vi "validate line configuration.vi"(7 "Module Config":refnum<class "Daqmx Module configuration.lvclass">, 11 "Mappings in":T1={"Line"={"Channel Array"=[], "Physical Channel"="", "Measurement Type"=enum."Digital Input", "Parameters"={"Digital Config"={"Invert Lines?"=FALSE}, "Voltage Config"={"Maximum Value (V)"=5.0, "Minimum Value (V)"=-5.0, "in terminal configuration (V)"=-1, "out terminal configuration (V)"=-1}, "Current Config"={"Maximum Value (A)"=0.02, "Minimum Value (A)"=0.0, "shunt resistor location"=-1, "input terminal configuration (C)"=-1, "external shunt resistor value"=249.0}, "RTD Config"={"Maximum Value (°C)"=100.0, "Minimum Value (°C)"=0.0, "resistance configuration"=2, "r0"=100.0, "current excitation value"=0.0025, "rtd type"=10137, "current excitation source"=10167}, "Thermocouple Config"={"Minimum Value (C)"=0.0, "Maximum Value (C)"=100.0, "thermocouple type"=10072, "cjc source"=10116, "cjc value"=25.0}, "Strain Config"={"Maximum Value"=0.001, "Minimum Value"=-0.001, "bridge information"={"strain configuration"=10183, "lead wire resistance"=0.0, "initial bridge voltage"=0.0, "voltage excitation source"=10200, "voltage excitation value"=2.5}, "strain gage information"={"gage factor"=2.0, "nominal gage resistance"=350.0, "poisson ratio"=0.3}}, "PWM Config"={"Idle State"=FALSE}}}, "Maps"=[]} {"Line"."Parameters"."Voltage Config"."out terminal configuration (V)" items=["Default"=-1, "RSE"=10083, "Differential"=10106, "Pseudodifferential"=12529]; "Line"."Parameters"."Voltage Config"."in terminal configuration (V)" items=["Default"=-1, "RSE"=10083, "NRSE"=10078, "Differential"=10106, "Pseudodifferential"=12529]; "Line"."Parameters"."Current Config"."shunt resistor location" items=["default"=-1, "Internal"=10200, "External"=10167]; "Line"."Parameters"."Current Config"."input terminal configuration (C)" items=["default"=-1, "RSE"=10083, "NRSE"=10078, "Differential"=10106, "Pseudodifferential"=12529]; "Line"."Parameters"."RTD Config"."resistance configuration" items=["2-Wire"=2, "3-Wire"=3, "4-Wire"=4]; "Line"."Parameters"."RTD Config"."rtd type" items=["Pt3750"=12481, "Pt3851"=10071, "Pt3911"=12482, "Pt3916"=10069, "Pt3920"=10053, "Pt3928"=12483, "Custom"=10137]; "Line"."Parameters"."RTD Config"."current excitation source" items=["Internal"=10200, "External"=10167, "None"=10230]; "Line"."Parameters"."Thermocouple Config"."thermocouple type" items=["J"=10072, "K"=10073, "N"=10077, "R"=10082, "S"=10085, "T"=10086, "B"=10047, "E"=10055]; "Line"."Parameters"."Thermocouple Config"."cjc source" items=["Built-In"=10200, "Constant Value"=10116, "Channel"=10113]; "Line"."Parameters"."Strain Config"."bridge information"."strain configuration" items=["Full Bridge I"=10183, "Full Bridge II"=10184, "Full Bridge III"=10185, "Half Bridge I"=10188, "Half Bridge II"=10189, "Quarter Bridge I"=10271, "Quarter Bridge II"=10272]; "Line"."Parameters"."Strain Config"."bridge information"."voltage excitation source" items=["Internal"=10200, "External"=10167, "None"=10230]}) -> (1 "valid?":bool, 2 "errors":string, 3 "Mappings out":T1={"Line"={"Channel Array"=[], "Physical Channel"="", "Measurement Type"=enum."Digital Input", "Parameters"={"Digital Config"={"Invert Lines?"=FALSE}, "Voltage Config"={"Maximum Value (V)"=5.0, "Minimum Value (V)"=-5.0, "in terminal configuration (V)"=-1, "out terminal configuration (V)"=-1}, "Current Config"={"Maximum Value (A)"=0.02, "Minimum Value (A)"=0.0, "shunt resistor location"=-1, "input terminal configuration (C)"=-1, "external shunt resistor value"=249.0}, "RTD Config"={"Maximum Value (°C)"=100.0, "Minimum Value (°C)"=0.0, "resistance configuration"=2, "r0"=100.0, "current excitation value"=0.0025, "rtd type"=10137, "current excitation source"=10167}, "Thermocouple Config"={"Minimum Value (C)"=0.0, "Maximum Value (C)"=100.0, "thermocouple type"=10072, "cjc source"=10116, "cjc value"=25.0}, "Strain Config"={"Maximum Value"=0.001, "Minimum Value"=-0.001, "bridge information"={"strain configuration"=10183, "lead wire resistance"=0.0, "initial bridge voltage"=0.0, "voltage excitation source"=10200, "voltage excitation value"=2.5}, "strain gage information"={"gage factor"=2.0, "nominal gage resistance"=350.0, "poisson ratio"=0.3}}, "PWM Config"={"Idle State"=FALSE}}}, "Maps"=[]} {"Line"."Parameters"."Voltage Config"."out terminal configuration (V)" items=["Default"=-1, "RSE"=10083, "Differential"=10106, "Pseudodifferential"=12529]; "Line"."Parameters"."Voltage Config"."in terminal configuration (V)" items=["Default"=-1, "RSE"=10083, "NRSE"=10078, "Differential"=10106, "Pseudodifferential"=12529]; "Line"."Parameters"."Current Config"."shunt resistor location" items=["default"=-1, "Internal"=10200, "External"=10167]; "Line"."Parameters"."Current Config"."input terminal configuration (C)" items=["default"=-1, "RSE"=10083, "NRSE"=10078, "Differential"=10106, "Pseudodifferential"=12529]; "Line"."Parameters"."RTD Config"."resistance configuration" items=["2-Wire"=2, "3-Wire"=3, "4-Wire"=4]; "Line"."Parameters"."RTD Config"."rtd type" items=["Pt3750"=12481, "Pt3851"=10071, "Pt3911"=12482, "Pt3916"=10069, "Pt3920"=10053, "Pt3928"=12483, "Custom"=10137]; "Line"."Parameters"."RTD Config"."current excitation source" items=["Internal"=10200, "External"=10167, "None"=10230]; "Line"."Parameters"."Thermocouple Config"."thermocouple type" items=["J"=10072, "K"=10073, "N"=10077, "R"=10082, "S"=10085, "T"=10086, "B"=10047, "E"=10055]; "Line"."Parameters"."Thermocouple Config"."cjc source" items=["Built-In"=10200, "Constant Value"=10116, "Channel"=10113]; "Line"."Parameters"."Strain Config"."bridge information"."strain configuration" items=["Full Bridge I"=10183, "Full Bridge II"=10184, "Full Bridge III"=10185, "Half Bridge I"=10188, "Half Bridge II"=10189, "Quarter Bridge I"=10271, "Quarter Bridge II"=10272]; "Line"."Parameters"."Strain Config"."bridge information"."voltage excitation source" items=["Internal"=10200, "External"=10167, "None"=10230]})   [LabVIEW 2015, in "DAQmx Module editor node.lvclass"]
doc: "This VI validates modifications to the table of lines and returns any errors as strings."
uses:
  DAQmx Module editor node.lvclass
  Mappings.ctl
  <vilib>/NI/Tag Bus Module Framework/channel/TBM channel.lvclass
  module/configuration/Line.ctl
  module/configuration/Measurement Type.ctl
  module/configuration/Parameters.ctl
  Map.ctl
  module/configuration/Daqmx Module configuration.lvclass
  <vilib>/NI/Tag Bus/tag/tag descriptor.lvclass/tag descriptor.ctl
  <vilib>/NI/Tag Bus/tag/read tag name.vi
  <vilib>/NI/Tag Bus/tag/read data type.vi
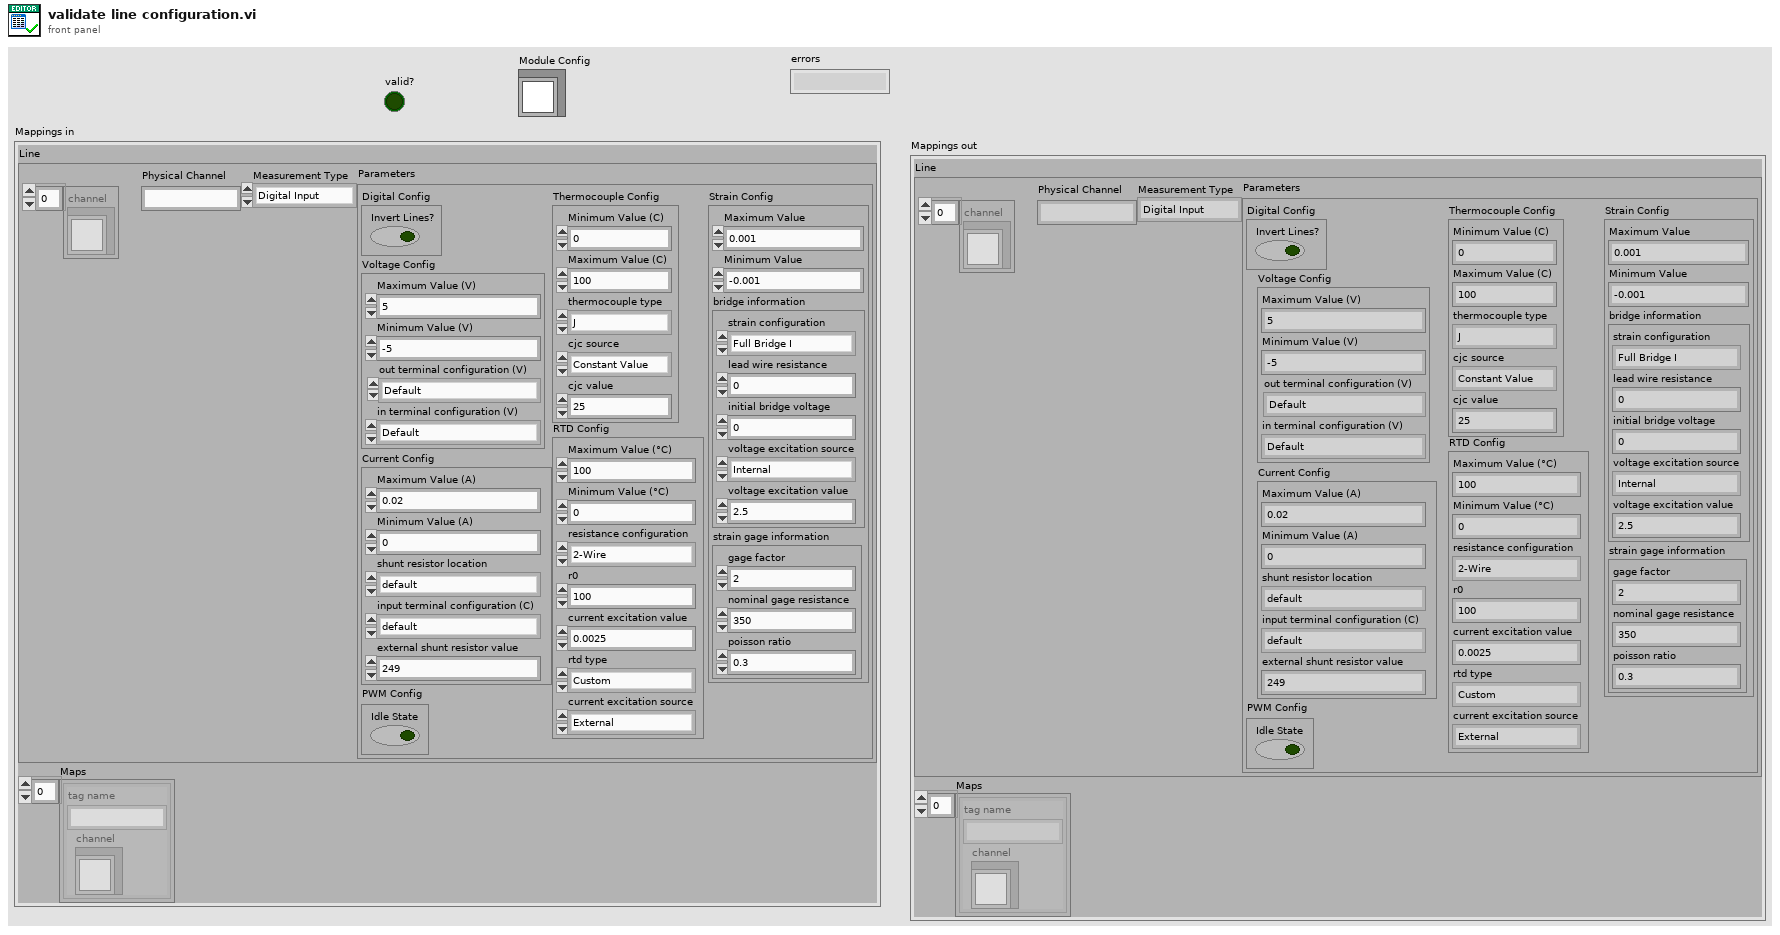
[diagram p1: front panel]
types:
  T1 = typedef "DAQmx Module editor node.lvclass/Mappings.ctl" = cluster{"Line":T2, "Maps":T5[]}
  T2 = typedef "DAQmx Module Configuration.lvclass/Line.ctl" = cluster{"Channel Array":refnum<class "TBM channel.lvclass">[], "Physical Channel":string, "Measurement Type":T3, "Parameters":T4}
  T3 = typedef "DAQmx Module Configuration.lvclass/Measurement Type.ctl" = enum16{"Digital Input", "Digital Output", "Voltage Input", "Voltage Output", "Current Input", "Current Output", "RTD", "Thermocouple", "Strain", "PWM"}
  T4 = typedef "DAQmx Module Configuration.lvclass/Parameters.ctl" = cluster{"Digital Config":cluster{"Invert Lines?":bool}, "Voltage Config":cluster{"Maximum Value (V)":dbl, "Minimum Value (V)":dbl, "in terminal configuration (V)":i32, "out terminal configuration (V)":i32}, "Current Config":cluster{"Maximum Value (A)":dbl, "Minimum Value (A)":dbl, "shunt resistor location":i32, "input terminal configuration (C)":i32, "external shunt resistor value":dbl}, "RTD Config":cluster{"Maximum Value (°C)":dbl, "Minimum Value (°C)":dbl, "resistance configuration":i32, "r0":dbl, "current excitation value":dbl, "rtd type":i32, "current excitation source":i32}, "Thermocouple Config":cluster{"Minimum Value (C)":dbl, "Maximum Value (C)":dbl, "thermocouple type":i32, "cjc source":i32, "cjc value":dbl}, "Strain Config":cluster{"Maximum Value":dbl, "Minimum Value":dbl, "bridge information":cluster{"strain configuration":i32, "lead wire resistance":dbl, "initial bridge voltage":dbl, "voltage excitation source":i32, "voltage excitation value":dbl}, "strain gage information":cluster{"gage factor":dbl, "nominal gage resistance":dbl, "poisson ratio":dbl}}, "PWM Config":cluster{"Idle State":bool}}
  T5 = typedef "DAQmx Module editor node.lvclass/Map.ctl" = cluster{"channel":refnum<class "TBM channel.lvclass">, "tag name":string}
  T6 = typedef "tag bus.lvlib/tag descriptor.lvclass/Data Type.ctl" = enum16{"Double", "Single", "I64", "I32", "I16", "I8", "U64", "U32", "U16", "U8", "Boolean", "String", "Array of Double", "Array of Single", "Array of I64", "Array of I32", "Array of I16", "Array of I8", "Array of U64", "Array of U32", "Array of U16", "Array of U8", "Array of Boolean", "Array of String"}
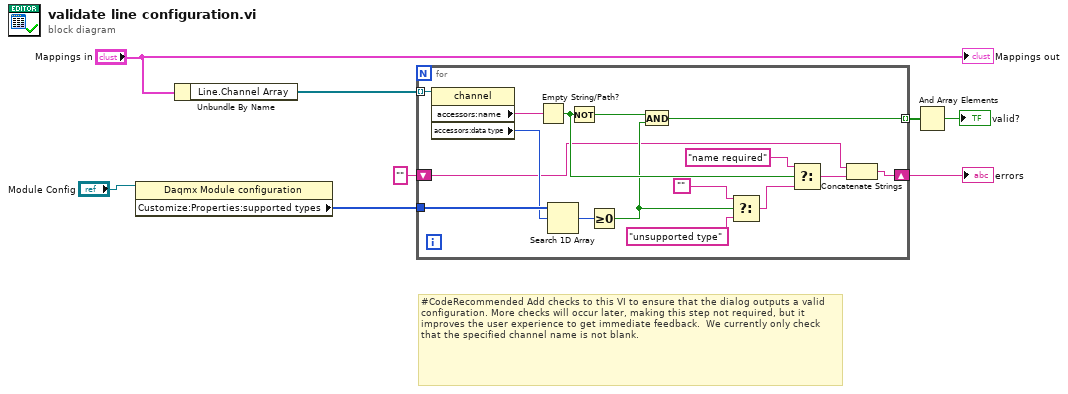
[diagram p0: block diagram]
diagram:
  # "#CodeRecommended Add checks to this VI to ensure that the dialog outputs a valid configuration. More checks will occur later, making this step not required, but it improves the user experience to get immediate feedback.  We currently only check that the specified channel name is not blank."
  n1 = property class="Daqmx Module configuration"(reference="Module Config") -> ("Customize:Properties:supported types"=w5:T6[])  [unwired: 1 in, 2 out]
  n2 = Unbundle By Name("Mappings in") -> ("Line.Channel Array"=w7:refnum<class "TBM channel.lvclass">[])
  n3 = for {
    tunnel: w7 -> [w24] mode=indexing
    tunnel: w5 -> [w21]
    tunnel: [w11] -> w3 mode=indexing
    shift-right: [w10] -> w4
    shift-left: "" -> [w9]
    n4 = property class="channel"(reference=w24) -> ("accessors:name"=w23:string, "accessors:data type"=w20:T6)  [unwired: 1 in, 2 out]
    n5 = Empty String/Path?(string/path=w23) -> (empty?=w18:bool)
    n6 = Search 1D Array(1D array=w21, element=w20) -> (index of element=w19:i32)  [unwired: 1 in]
    n7 = Not(x=w18) -> (.not. x?=w22:bool)
    n8 = Greater Or Equal To 0?(x=w19) -> (x >= 0?=w15:bool)
    n9 = And(x=w22, y=w15) -> (x .and. y?=w11:bool)
    n10 = Select(t="", s=w15, f="unsupported type") -> (s? t:f=w13:string)
    n11 = Select(t="name required", s=w18, f=w13) -> (s? t:f=w16:string)
    n12 = Concatenate Strings(w9, w16) -> (w10:string)
  }
  "errors" <- w4
  n13 = And Array Elements(Boolean array=w3) -> (logical AND=→"valid?":bool)
  "Mappings out" <- "Mappings in"
